vi "Smooth_example.vi"() -> ()   [LabVIEW 2023, in "ELTA.lvlib"]
uses:
  ELTA.lvlib
  <vilib>/Utility/file.llb/Read Delimited Spreadsheet (string).vi
panel:
  out "Smooth_order_2":cluster{"X":dbl, "Y":dbl}[](graph)
  out "Vince Test":cluster{"X":dbl, "Y":dbl}[](graph)
  in  "file path":path=path "C:/Users/Vince_Wu/Desktop/SA_inPhase_Example/DualCh_20241107_180730_72_forELTA.csv"
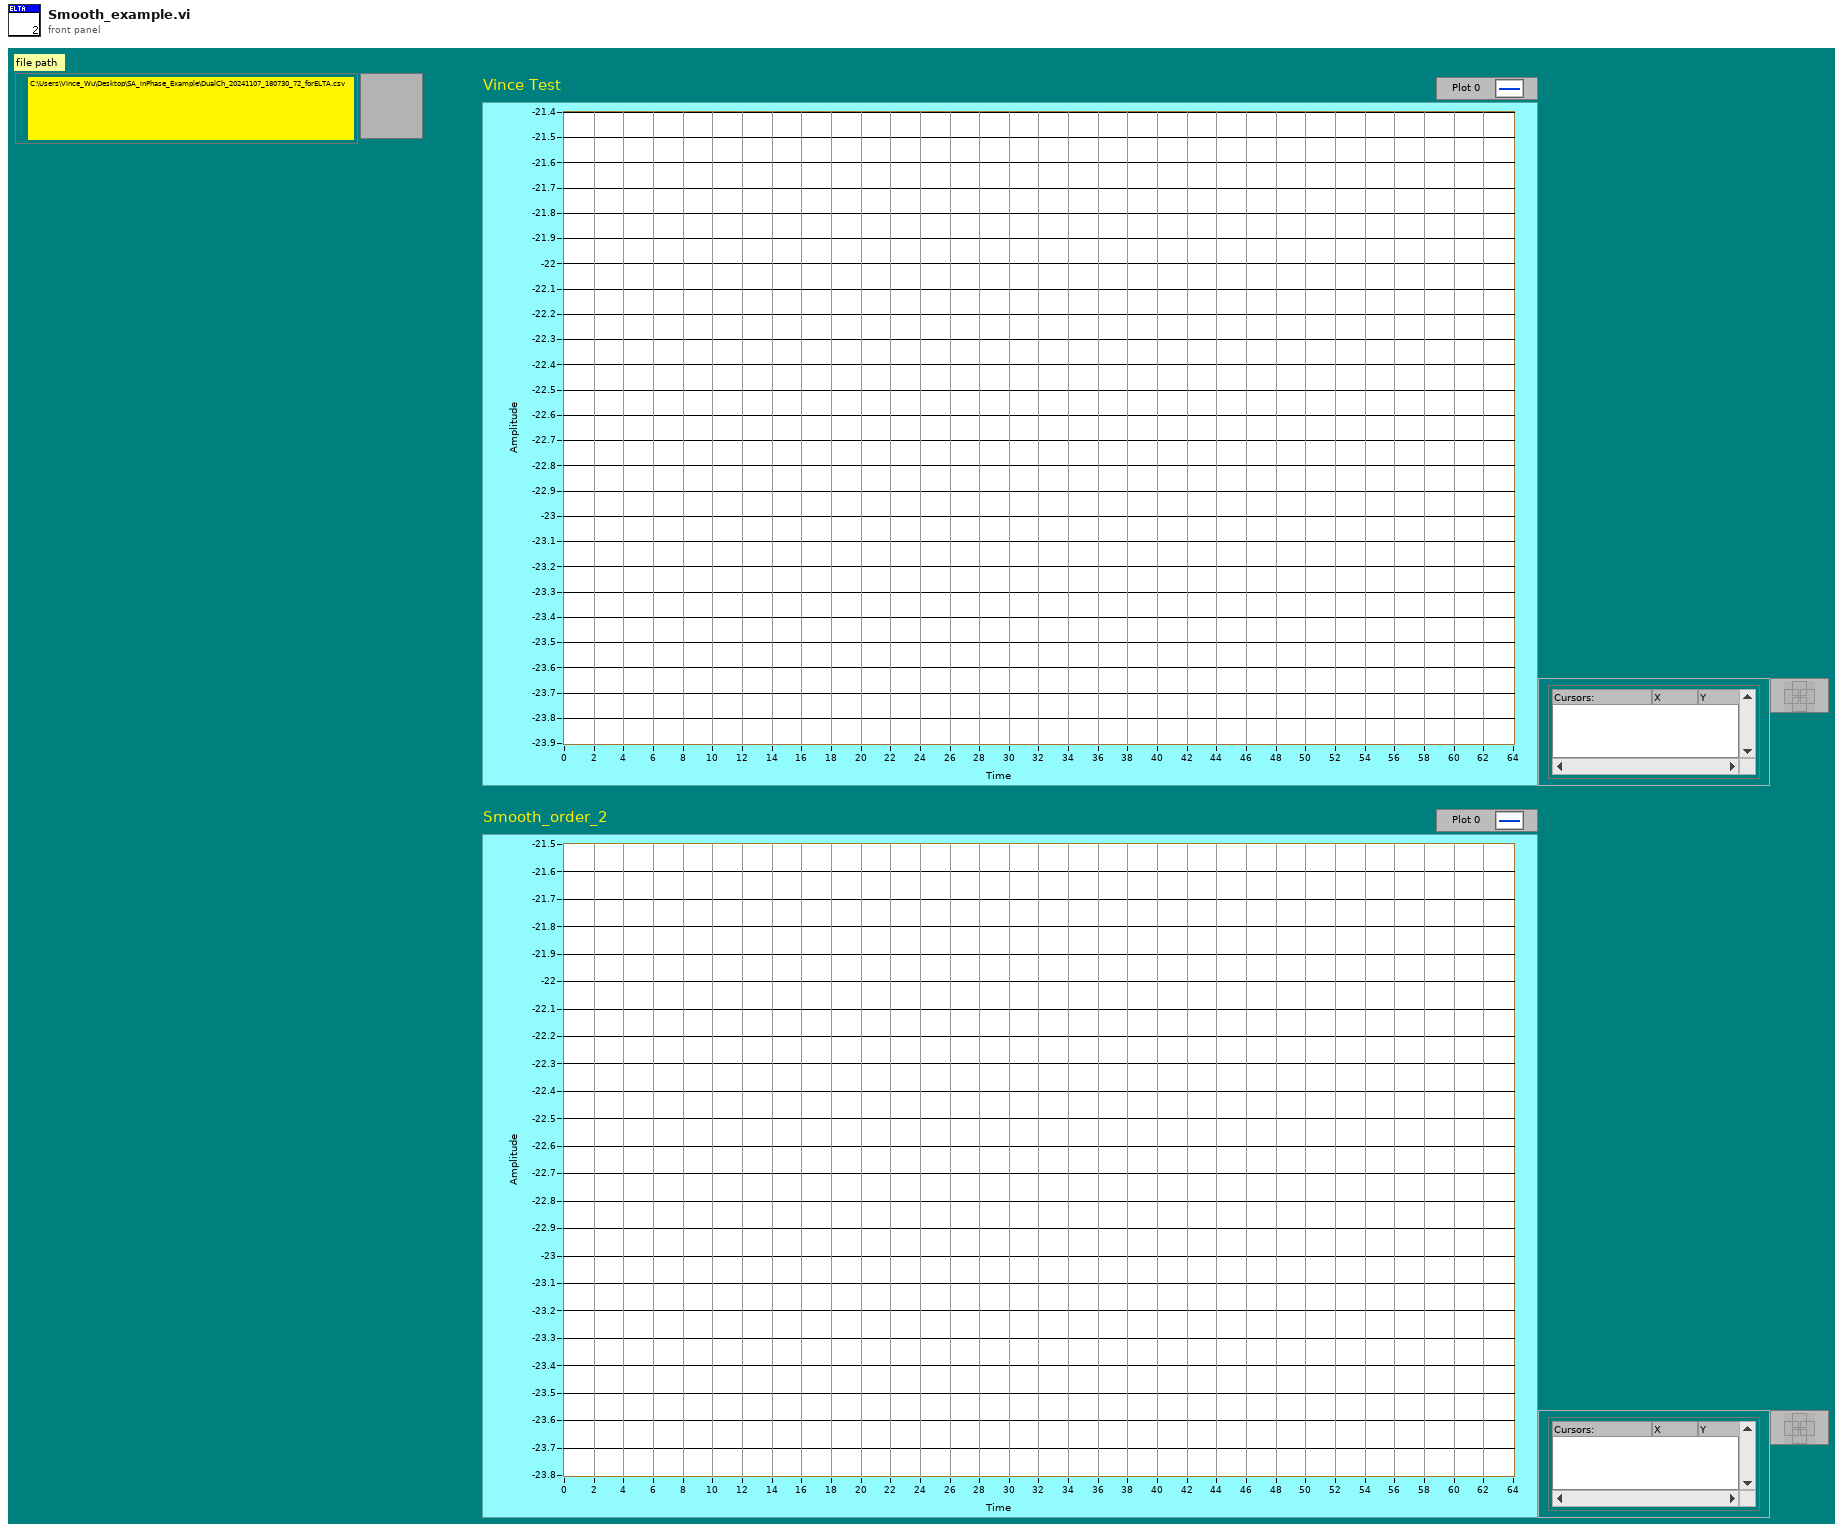
[diagram p1: front panel]
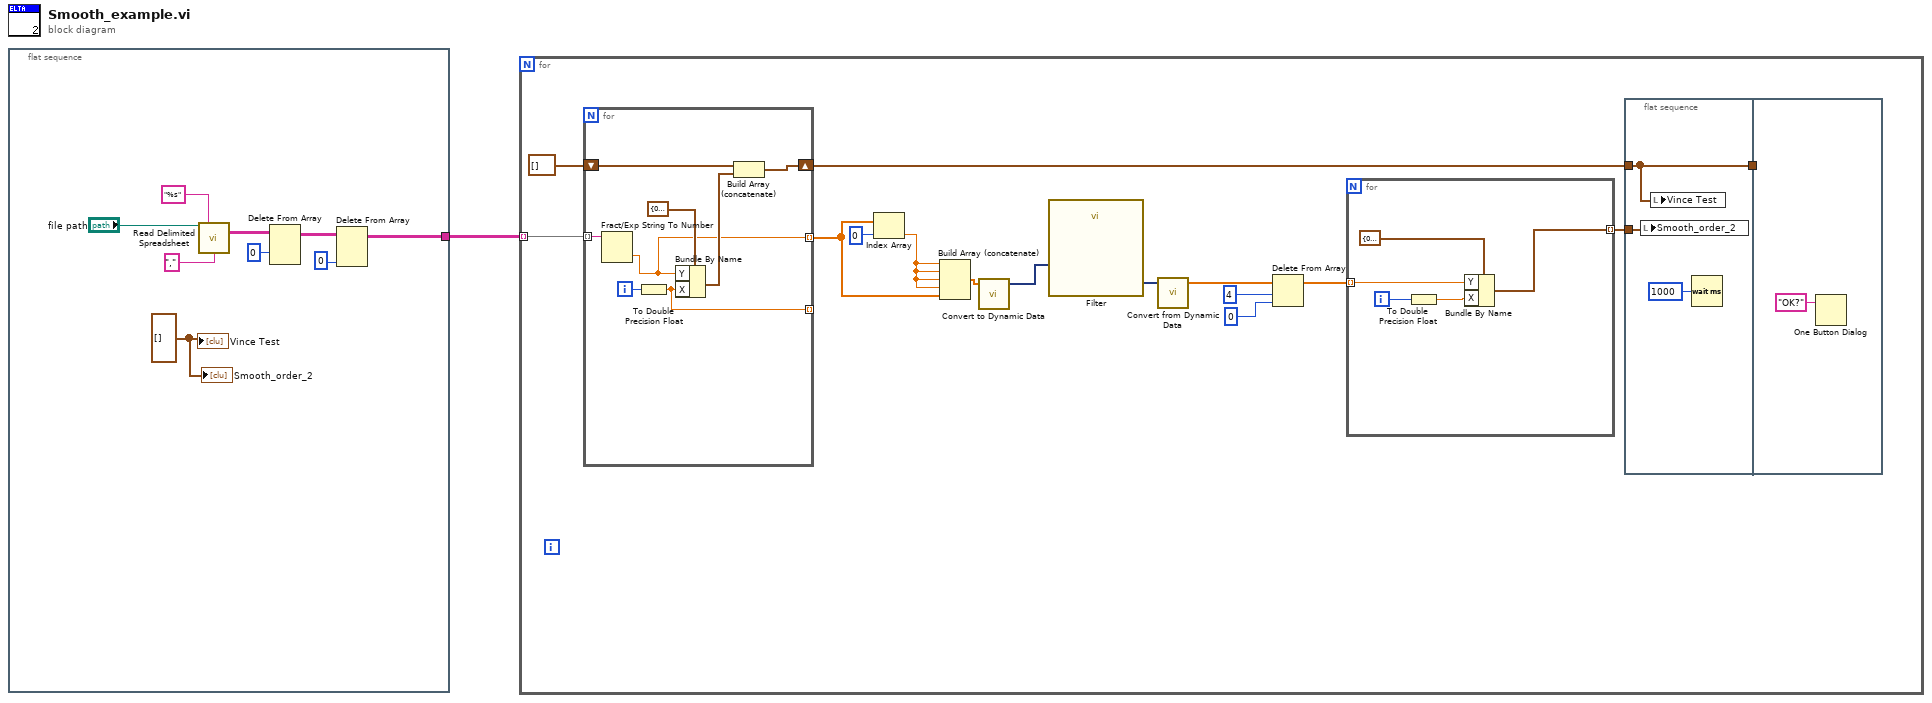
[diagram p0: block diagram]
diagram:
  n1 = flat-sequence {
    tunnel: [w3] -> w1
    frame #0 {
      w2 = cluster{"X":dbl, "Y":dbl}[] [] ("XY Graph")
      n2 = call-poly <vilib>:"Read Delimited Spreadsheet.vi"("file path (dialog if empty)"="file path", "format (%s)"="%s" ("format (%.3f)"), "delimiter (\\t)"="," ("delimiter (\\t)")) -> ("all rows"=w8:string[][])  [unwired: 7 in, 5 out]
      n3 = Delete From Array(array=w8, index (row)=0) -> (array with subset deleted=w4:string[][])  [unwired: 2 in, 1 out]
      n4 = Delete From Array(array=w4, index (col)=0 ("index (row)")) -> (array with subset deleted=w3:string[][])  [unwired: 2 in, 1 out]
      "Vince Test" <- w2
      "Smooth_order_2" <- w2
    }
  }
  n5 = for {
    tunnel: w1 -> [w25] mode=indexing
    n6 = for {
      tunnel: w25 -> [w41] mode=indexing
      shift-right: [w38] -> w22
      shift-left: cluster{"X":dbl, "Y":dbl}[] [] ("XY Graph") -> [w40]
      tunnel: [w36] -> w17 mode=indexing
      tunnel: [w35] -> _ mode=indexing
      i -> [w37]
      n7 = Fract/Exp String To Number(string=w41) -> (number=w36:dbl)  [unwired: 3 in, 1 out]
      n8 = To Double Precision Float(number=w37) -> (double precision float=w35:dbl)
      n9 = Bundle By Name(cluster=cluster{"X":dbl, "Y":dbl} {"X"=0.0, "Y"=0.0} ("element"), "Y"=w36, "X"=w35) -> (w39:cluster{"X":dbl, "Y":dbl})
      n10 = Build Array (concatenate)(w40, w39) -> (w38:cluster{"X":dbl, "Y":dbl}[])
    }
    n11 = Index Array(array=w17, index=0) -> (element=w11:dbl)
    n12 = Build Array (concatenate)(w11, w11, w11, w11, w17) -> (w15:dbl[])
    n13 = call "Convert to Dynamic Data"("Array"=w15) -> ("Dynamic Data Type"=w21:dynamicdata)  [unwired: 3 in]
    n14 = call "Filter"("Signal"=w21) -> ("Filtered Signal"=w20:dynamicdata)  [unwired: 9 in, 1 out]
    n15 = call "Convert from Dynamic Data"("Dynamic Data Type"=w20) -> ("Array"=w19:dbl[])  [unwired: 3 in]
    n16 = Delete From Array(array=w19, length=4, index=0) -> (array with subset deleted=w14:dbl[])  [unwired: 1 out]
    n17 = for {
      tunnel: w14 -> [w29] mode=indexing
      tunnel: [w26] -> w18 mode=indexing
      i -> [w27]
      n18 = To Double Precision Float(number=w27) -> (double precision float=w28:dbl)
      n19 = Bundle By Name(cluster=cluster{"X":dbl, "Y":dbl} {"X"=0.0, "Y"=0.0} ("element"), "Y"=w29, "X"=w28) -> (w26:cluster{"X":dbl, "Y":dbl})
    }
    n20 = flat-sequence {
      tunnel: w22 -> [w32]
      tunnel: [w32] -> w24
      tunnel: w18 -> [w31]
      tunnel: w24 -> [_]
      frame #0 {
        n21 = local write "Smooth_order_2"(w31) -> ()
        n22 = local write "Vince Test"(w32) -> ()
        n23 = Wait (ms)(milliseconds to wait=u32 1000) -> ()  [unwired: 1 out]
      }
      frame #1 {
        n24 = One Button Dialog(message="OK?") -> ()  [unwired: 1 in, 1 out]
      }
    }
  }
